vi "PTSequencer.form DIM subscriptions.vi"(0 "DIM subsriptions":string[](array[string]), 1 "conditions":T4[](array[typedef]), 2 "used subsriptions in":string[](array[string]), 4 "trendmsgs in":T1[](array[typedef])) -> (14 "DIM subsriptions out":string[](array[string]), 16 "used subsriptions out":string[](array[string]), 18 "trendmsgs out":T1[](array[typedef]))   [LabVIEW 2014, in "PTSequencer.lvlib"]
uses:
  PTSequencer.lvlib
  PTSequencer.DIM service condition.ctl
  CS_Core/CSSystem/CoreDefs/CoreDefs.rawDataType.ctl
  CS_Core/BaseProcess/BaseProcess.event definition.ctl
  CS_Core/CAEObj/CAEObj.event definition.ctl
  CS_Core/BaseProcess/BaseProcess.descriptor string definition.ctl
  CS_Core/BaseProcess/BaseProcess.lvlib
  CS_Core/CAEObj/CAEObj.lvlib
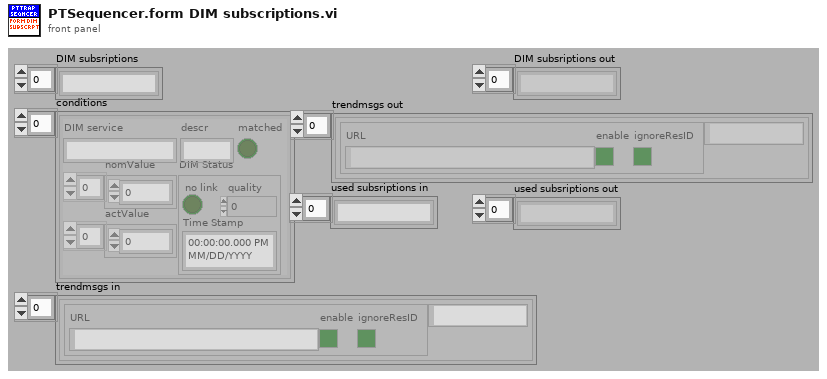
[diagram p1: front panel]
types:
  T1 = typedef "BaseProcess.lvlib/BaseProcess.event definition.ctl" = cluster{"CAEEvtDef":T2, "Data Descriptor":T3}
  T2 = typedef "CAEObj.lvlib/CAEObj.event definition.ctl" = cluster{"URL":string, "enable":bool, "ignoreResID":bool}
  T3 = typedef "BaseProcess.lvlib/BaseProcess.descriptor string definition.ctl" = string
  T4 = typedef "PTSequencer.lvlib/PTSequencer.DIM service condition.ctl" = cluster{"DIM service":string, "descr":string, "nomValue":T5, "actValue":T5, "matched":bool, "DIM Status":cluster{"no link":bool, "quality":i32, "Time Stamp":timestamp}}
  T5 = typedef "CoreDefs.rawDataType.ctl" = i8[]
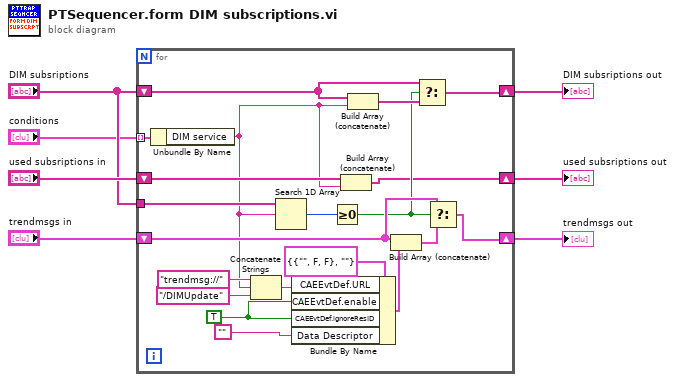
[diagram p0: block diagram]
diagram:
  n1 = for {
    tunnel: "DIM subsriptions" -> [w20]
    shift-right: [w15] -> w2
    shift-left: "trendmsgs in" -> [w19]
    shift-right: [w17] -> w4
    shift-left: "DIM subsriptions" -> [w8]
    tunnel: "conditions" -> [w12] mode=indexing
    shift-right: [w9] -> w1
    shift-left: "used subsriptions in" -> [w11]
    w26 = TRUE ("CAEEvtDef.ignoreResID")
    n2 = Unbundle By Name(w12) -> ("DIM service"=w10:string)
    n3 = Concatenate Strings("trendmsg://", w10, "/DIMUpdate" ("string")) -> (w23:string)
    n4 = Search 1D Array(1D array=w20, element=w10) -> (index of element=w13:i32)  [unwired: 1 in]
    n5 = Bundle By Name(cluster=T1 {"CAEEvtDef"={"URL"="", "enable"=FALSE, "ignoreResID"=FALSE}, "Data Descriptor"=""} ("event definition"), "CAEEvtDef.URL"=w23, "CAEEvtDef.enable"=w26, "CAEEvtDef.ignoreResID"=w26, "Data Descriptor"="") -> (w21:T1)
    n6 = Greater Or Equal To 0?(x=w13) -> (x >= 0?=w14:bool)
    n7 = Build Array (concatenate)(w11, w10) -> (w9:string[])
    n8 = Build Array (concatenate)(w8, w10) -> (w16:string[])
    n9 = Build Array (concatenate)(w19, w21) -> (w18:T1[])
    n10 = Select(t=w8, s=w14, f=w16) -> (s? t:f=w17:string[])
    n11 = Select(t=w19, s=w14, f=w18) -> (s? t:f=w15:T1[])
  }
  "DIM subsriptions out" <- w4
  "trendmsgs out" <- w2
  "used subsriptions out" <- w1
